vi "Q Loop.vi"(10 "Q":refnum<queue>) -> ()   [LabVIEW 2021, in "Q Async.lvlib"]
uses:
  Q Async.lvlib
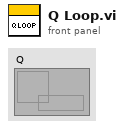
[diagram p1: front panel]
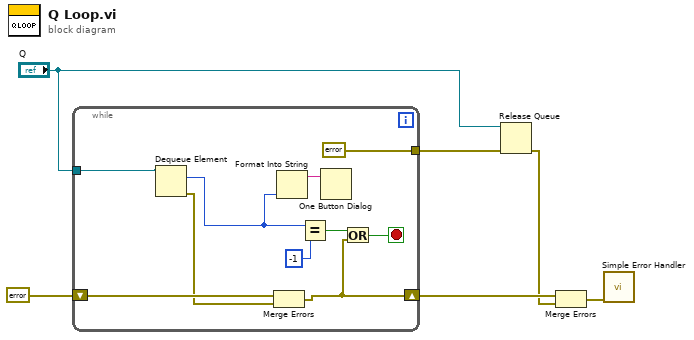
[diagram p0: block diagram]
diagram:
  n1 = while {
    tunnel: "Q" -> [w7]
    shift-right: [w8] -> w5
    shift-left: errorcluster {"status"=FALSE, "code"=0, "source"=""} ("error IO") -> [w14]
    tunnel: [errorcluster {"status"=FALSE, "code"=0, "source"=""} ("error in (no error)")] -> w2
    stop <- w9 stop-if-true
    n2 = Dequeue Element(queue=w7) -> (element=w11:i32, error out=w13:errorcluster)  [unwired: 2 in, 2 out]
    n3 = Merge Errors(w14, w13) -> (w8:errorcluster)
    n4 = Format Into String(w11) -> (resulting string=w12:string)  [unwired: 3 in, 1 out]
    n5 = Equal?(x=w11, y=-1) -> (x = y?=w16:bool)
    n6 = One Button Dialog(message=w12) -> ()  [unwired: 1 in, 1 out]
    n7 = Or(x=w16, y=w8) -> (x .or. y?=w9:bool)
  }
  n8 = Release Queue(queue="Q", error in (no error)=w2) -> (error out=w3:errorcluster)  [unwired: 1 in, 2 out]
  n9 = Merge Errors(w5, w3) -> (w4:errorcluster)
  n10 = call <vilib>:"Simple Error Handler.vi"("error in (no error)"=w4) -> ()  [unwired: 4 in, 5 out]
